vi "detectISOSPI.vi"(8 "errin":errorcluster) -> (0 "sortie d'erreur":errorcluster caption="errout", 3 "cas faux":string)   [LabVIEW 2020]
uses:
  <vilib>/Instr/_visa.llb/VISA Find Search Mode.ctl
  <vilib>/Instr/_visa.llb/VISA Configure Serial Port (Instr).vi
panel:
  out "buffer de lecture":string
  # "2A49 444E 3F0A"
  # "*IDN?"
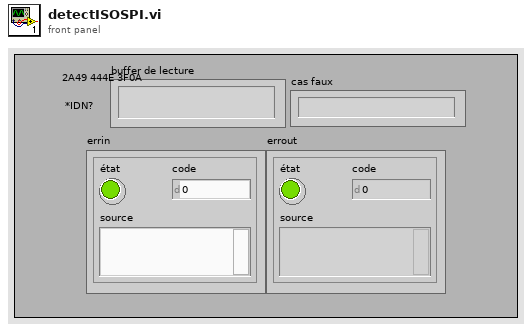
[diagram p1: front panel]
types:
  T1 = typedef "VISA Find Search Mode.ctl" = u32
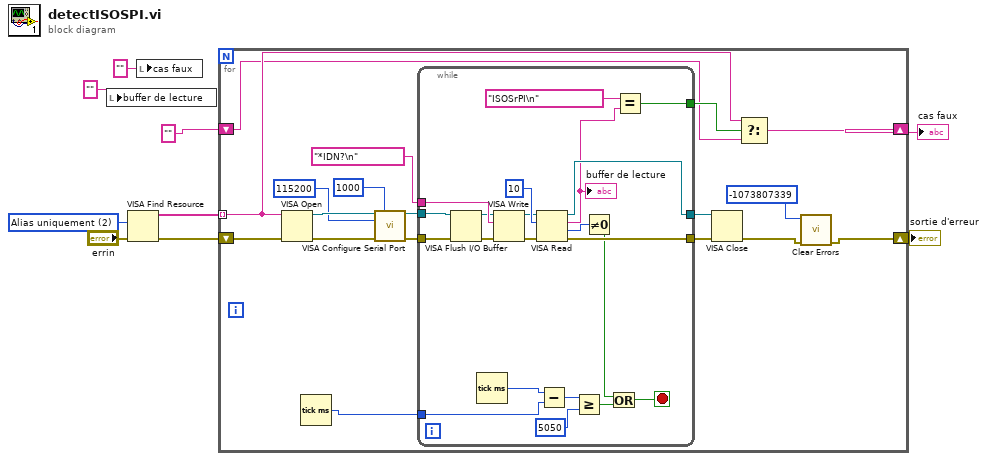
[diagram p0: block diagram]
diagram:
  w1 = T1 2 items=["Noms canoniques uniquement"=0, "Alias uniquement"=2, "Inclure les alias correspondants"=3, "Inclure tous les alias"=4] ("Search Mode")
  n1 = local write "buffer de lecture"("" ("buffer de lecture")) -> ()
  n2 = VISA Find Resource(8:"errin", 10:w1) -> (0:w8:errorcluster, 3:w7:string[])  [unwired: 1 in, 1 out]
  n3 = local write "cas faux"("" ("cas faux")) -> ()
  n4 = for {
    tunnel: w7 -> [w16] mode=indexing
    shift-right: [w12] -> w9
    shift-left: w8 -> [w18]
    shift-right: [w15] -> w5
    shift-left: "" ("cas faux") -> [w14]
    n5 = VISA Open(error in (no error)=w18, VISA resource name=w16) -> (VISA resource name=w26:refnum<visa-resource-name>, error out=w25:errorcluster)  [unwired: 3 in]
    n6 = Tick Count (ms)() -> (millisecond timer value=w10:u32)
    n7 = call-poly "VISA Configure Serial Port"("VISA resource name"=w26, "timeout (10sec)"=u32 1000, "baud rate (9600)"=u32 115200, "error in (no error)"=w25) -> ("VISA resource name out"=w21:refnum<visa-resource-name>, "error out"=w23:errorcluster)  [unwired: 10 in]
    n8 = while {
      tunnel: [w48] -> w27
      tunnel: w23 -> [w40]
      tunnel: "*IDN?\n" ("buffer d'écriture") -> [w45]
      tunnel: w21 -> [w41]
      tunnel: [w43] -> w20
      tunnel: [w35] -> w17
      tunnel: w10 -> [w33]
      stop <- w28 stop-if-true
      n9 = VISA Flush I/O Buffer(VISA resource name=w41, error in (no error)=w40) -> (VISA resource name out=w38:refnum<visa-resource-name>, error out=w39:errorcluster)  [unwired: 1 in]
      n10 = Tick Count (ms)() -> (millisecond timer value=w34:u32)
      n11 = VISA Write(VISA resource name=w38, write buffer=w45, error in (no error)=w39) -> (VISA resource name out=w42:refnum<visa-resource-name>, error out=w44:errorcluster)  [unwired: 1 out]
      n12 = VISA Read(VISA resource name=w42, byte count=u32 10 ("nombre d'octets"), error in (no error)=w44) -> (VISA resource name out=w43:refnum<visa-resource-name>, read buffer=w37:string, return count=w46:u32, error out=w48:errorcluster)
      "buffer de lecture" <- w37
      n13 = Subtract(x=w34, y=w33) -> (x-y=w32:u32)
      n14 = Greater Or Equal? ("Supérieur ou égal ?")(x=w32, y=u32 5050) -> (x >= y?=w30:bool)
      n15 = Not Equal To 0?(x=w46) -> (x != 0?=w29:bool)
      n16 = Or(x=w29, y=w30) -> (x .or. y?=w28:bool)
      n17 = Equal? ("Égaux ?")(x="ISOSrPI\n", y=w37) -> (x = y?=w35:bool)
    }
    n18 = VISA Close(VISA resource name=w20, error in (no error)=w27) -> (error out=w13:errorcluster)
    n19 = Select ("Sélectionner")(t=w16, s=w17, f=w14) -> (s? t:f=w15:string)
    n20 = call <vilib>:"Clear Errors.vi"("error in (no error)"=w13, "specific error code to clear (0: all)"=-1073807339) -> ("error out"=w12:errorcluster)  [unwired: 4 in, 1 out]
  }
  "sortie d'erreur" <- w9
  "cas faux" <- w5
